vi "UPRcontroller_v00_basedonlsmv66.vi"() -> ()   [LabVIEW 2015] (continued)
                            n907 = call "eraseCI_img.vi"() -> ()  [unwired: 12 in]
                            n908 = call "eraseAI_img.vi"() -> ()  [unwired: 12 in]
                          }
                          frame "Lifetime (scan)" {
                            n909 = disable-structure shown="Disabled" {
                              disable-tunnel: w3434 -> [w3435 _]
                              frame Disabled {
                                n910 = stacked-sequence {
                                tunnel: w3435 -> [_ _ w3449 _ _]
                                frame #0 {
                                n911 = disable-structure shown="Disabled" {
                                frame Disabled {
                                n912 = call "stoperaseCI.vi"() -> ()  [unwired: 12 in]
                                n913 = call "stoperaseDO_img.vi"() -> ()  [unwired: 12 in]
                                n914 = call "stoperaseAO_img.vi"() -> ()  [unwired: 12 in]
                                n915 = call "stoperaseAI_img.vi"() -> ()  [unwired: 12 in]
                                }
                                frame Enabled {
                                }
                                }
                                }
                                frame #1 {
                                n916 = disable-structure shown="Disabled" {
                                frame Disabled {
                                n917 = local read "Acquisition time"() -> (w3439:i32)
                                n918 = call "collect_allLT_img.vi"() -> ("counts"=w3441:i32)  [unwired: 1 out]
                                n919 = local read "counts"() -> (w3442:i32)
                                n920 = Add(x=w3442, y=w3441) -> (x+y=w3440:i32)
                                "counts" <- w3440
                                n921 = Divide(x=w3440, y=w3439) -> (x/y=w3438:dbl)
                                n922 = Multiply(x=1000.0, y=w3438) -> (x*y=w3437:dbl)
                                n923 = local write "Avg Counts/s"(w3437) -> ()
                                }
                                frame Enabled {
                                }
                                }
                                }
                                frame #2 {
                                w3445 = u16 0 items=["Stream to disk", "Post process", "real time process"] ("Ring")
                                n924 = local read "T3R Data processing"() -> (w3444:u16)
                                n925 = local read "save\ndata"() -> (w3447:bool)
                                n926 = Equal?(x=w3444, y=w3445) -> (x = y?=w3443:bool)
                                n927 = Not(x=w3443) -> (.not. x?=w3448:bool)
                                n928 = And(x=w3447, y=w3448) -> (x .and. y?=w3446:bool)
                                n929 = case shown="True" w3446 {
                                tunnel: w3449 -> [_ w3451]
                                frame False {
                                }
                                frame True {
                                n930 = local read "filename prefix"() -> (w3452:string)
                                n931 = local read "data dir"() -> (w3457:path)
                                n932 = call "2pparameters.vi"("command"="get") -> ("params out"=w3472:T12)  [unwired: 1 in]
                                n933 = call "generatedatafilename.vi"("timestamp"=w3451, "filename prefix in"=w3452) -> ("full-filename"=w3450:string)
                                n934 = Unbundle By Name(w3472) -> ("srate"=w3470:sgl, "sAOxy"=w3469:i32, "Xpixels Img"=w3467:i32, "Ypixels Img"=w3465:i32)
                                n935 = Concatenate Strings(w3450, ".lvpt3img" ("string")) -> (w3455:string)
                                n936 = Build Path(base path=w3457, name or relative path=w3455) -> (appended path=w3454:path)
                                n937 = To Unsigned Long Integer(number=w3470) -> (unsigned 32bit integer=w3471:u32)
                                n938 = To Unsigned Long Integer(number=w3469) -> (unsigned 32bit integer=w3468:u32)
                                n939 = To Unsigned Long Integer(number=w3467) -> (unsigned 32bit integer=w3466:u32)
                                n940 = To Unsigned Long Integer(number=w3465) -> (unsigned 32bit integer=w3464:u32)
                                n941 = call "PH-temp-raw.vi"("command"="get") -> ("array out"=w3463:u32[])  [unwired: 1 in]
                                n942 = Build Array (concatenate)(w3471, w3468, w3466, w3464, w3463) -> (w3462:u32[])
                                n943 = Open/Create/Replace File(file path (use dialog)=w3454, operation (0:open)=T9."replace or create") -> (refnum out=w3461:refnum<file>, error out=w3460:errorcluster)  [unwired: 4 in, 1 out]
                                n944 = Write to Binary File(file (use dialog)=w3461, data=w3462, error in=w3460, 5:FALSE ("prepend array or string size? (T)")) -> (refnum out=w3458:refnum<file>, error out=w3459:errorcluster)  [unwired: 2 in, 1 out]
                                n945 = Close File(refnum=w3458, error in=w3459) -> ()  [unwired: 2 out]
                                }
                                }
                                n946 = call "stoperaseLT_img.vi"() -> ()  [unwired: 1 in]
                                }
                                frame #3 {
                                w3478 = u16 1 items=["Stream to disk", "Post process", "real time process"] ("Ring")
                                n947 = local read "T3R Data processing"() -> (w3477:u16)
                                n948 = Equal?(x=w3477, y=w3478) -> (x = y?=w3476:bool)
                                n949 = case shown="True" w3476 {
                                frame False {
                                }
                                frame True {
                                # "intensity"
                                # "lifetime"
                                # "intensity"
                                n950 = property on="img_CH1" class="IntGraph (strict)"() -> ("Value"=w3491:sgl[][])  [unwired: 2 in, 2 out]
                                n951 = Array Max & Min(array=w3491) -> (max value=w3492:sgl)  [unwired: 3 out]
                                n952 = local read "lineshift"() -> (w3479:i32)
                                n953 = local read "min phot"() -> (w3493:u32)
                                n954 = To Unsigned Long Integer(number=w3492) -> (unsigned 32bit integer=w3495:u32)
                                n955 = local read "counts"() -> (w3481:i32)
                                n956 = call "wrapcutlifetime.vi"("lineshift"=w3479) -> ("pt3img"=w3490:u16[][], "lifetimes"=w3488:sgl[][], "okay"=w3483:bool, "# of frames"=w3480:i32)
                                "frames recorded" <- w3480
                                n957 = Greater?(x=w3493, y=w3495) -> (0:w3494:bool)
                                n958 = Quotient & Remainder(x=w3481, y=w3480) -> (floor(x/y)=w3482:i32)  [unwired: 1 out]
                                n959 = Transpose 2D Array(2D array=w3490) -> (transposed array=w3484:u16[][])
                                n960 = Transpose 2D Array(2D array=w3488) -> (transposed array=w3489:sgl[][])
                                n961 = And(x=w3494, y=w3483) -> (x .and. y?=w3496:bool)
                                n962 = local write "img_CH2"(w3489) -> ()
                                n963 = local write "photons/frame"(w3482) -> ()
                                n964 = Array Max & Min(array=w3484) -> (max value=w3485:u16)  [unwired: 3 out]
                                n965 = To Single Precision Float(number=w3484) -> (single precision float=w3487:sgl[][])
                                n966 = case shown="True" w3496 {
                                tunnel: w3495 -> [_ w3500]
                                frame False {
                                }
                                frame True {
                                n967 = Quotient & Remainder(x=w3500, y=u32 2 ("min phot")) -> (floor(x/y)=w3499:u32)  [unwired: 1 out]
                                n968 = Max & Min(x=w3499, y=u32 5) -> (max(x,y)=w3498:u32)  [unwired: 1 out]
                                n969 = local write "min phot"(w3498) -> ()
                                }
                                }
                                n970 = To Double Precision Float(number=w3485) -> (double precision float=w3486:dbl)
                                n971 = local write "img_CH1"(w3487) -> ()
                                n972 = property on="img_CH1" class="IntGraph (strict)"("ZScale.Maximum"=w3486) -> ()  [unwired: 2 in, 2 out]
                                }
                                }
                                }
                                frame #4 {
                                w3504 = u16 1 items=["Stream to disk", "Post process", "real time process"] ("Ring")
                                n973 = local read "T3R Data processing"() -> (w3503:u16)
                                n974 = Equal?(x=w3503, y=w3504) -> (x = y?=w3502:bool)
                                n975 = case shown="False" w3502 {
                                frame False {
                                # "intensity"
                                n976 = local read "Current Average"() -> (w3509:sgl)
                                n977 = local read "image2list"() -> (w3505:u16)
                                n978 = local read "image1list"() -> (w3506:u16)
                                n979 = call "dattoimage.vi"("image2list"=w3505, "Current Average"=w3509, "image1list"=w3506) -> ("image 1 array out"=w3508:sgl[][])  [unwired: 1 out]
                                n980 = Transpose 2D Array(2D array=w3508) -> (transposed array=w3507:sgl[][])
                                n981 = local write "img_CH2"(w3507) -> ()
                                }
                                frame True {
                                }
                                }
                                }
                                }
                              }
                              frame Enabled {
                              }
                            }
                          }
                        }
                        n982 = local write "64bit disabled"(TRUE ("64bit disabled")) -> ()
                      }
                      frame #9 {
                        # "Reset the AO values after scanning to a known state (possibly source of delay after pressing stop)"
                        n983 = call "2pparameters.vi"("command"="get") -> ("params out"=w3514:T12)  [unwired: 1 in]
                        n984 = Unbundle By Name(w3514) -> ("auto OD"=w3513:bool, "autoshutter"=w3511:bool, "aAS"=w3510:u32[])
                        n985 = case shown="True" w3513 {
                          frame False {
                          }
                          frame True {
                            n986 = call "configuration.vi"("command"="get") -> ("config out"=w3519:T14)  [unwired: 2 in, 1 out]
                            n987 = call "2pparameters.vi"("command"="get") -> ("params out"=w3522:T12)  [unwired: 1 in]
                            n988 = Unbundle By Name(w3519) -> ("image OD"=w3517:u16)
                            n989 = Unbundle By Name(w3522) -> ("ODfilt"=w3518:u16)
                            n990 = call "filterwheelcontrol_nothorlabslib.vi"("Current OD filt"=w3517, "New ODfilt"=w3518) -> ()  [unwired: 1 in]
                          }
                        }
                        n991 = case shown="True" w3511 {
                          tunnel: w3510 -> [_ w3515]
                          frame False {
                          }
                          frame True {
                            n992 = call "shuttercontrol_multi.vi"("Autoshutter Chans"=w3515, "command"="close") -> ()  [unwired: 1 in, 1 out]
                          }
                        }
                        n993 = disable-structure shown="Disabled" {
                          frame Disabled {
                            # "<- possible source of delay"
                            n994 = call "reset AO_DO_v3.vi"() -> ()  [unwired: 12 in]
                          }
                          frame Disabled {
                            # "<- possible source of delay"
                            n995 = call "reset AO_DO_v3.vi"() -> ()  [unwired: 12 in]
                          }
                          frame Enabled {
                          }
                        }
                        n996 = flat-sequence {
                          frame #0 {
                            n997 = call "reset AO_DO_v3.vi"() -> ()  [unwired: 12 in]
                          }
                          frame #1 {
                            n998 = call "stoperaseCI.vi"() -> ()  [unwired: 12 in]
                            n999 = call "stoperaseDO_img.vi"() -> ()  [unwired: 12 in]
                            n1000 = call "stoperaseAO_img.vi"() -> ()  [unwired: 12 in]
                            n1001 = call "stoperaseAI_img.vi"() -> ()  [unwired: 12 in]
                          }
                        }
                      }
                      frame #10 {
                        # "CI: counter input (for photon counting)"
                        # "If waveform determined scan... separates out scanning waveforms from 'waveform generation' waveforms"
                        n1002 = stacked-sequence {
                          tunnel: w3536 -> [w3539 _ _ _ _ _]
                          tunnel: w3535 -> [w3538 _ _ _ _ _]
                          tunnel: w3534 -> [w3537 _ _ _ _ _]
                          tunnel: w3533 -> [_ w3588 _ _ _ _]
                          tunnel: w3532 -> [_ w3587 w3642 w3761 _ _]
                          tunnel: w3531 -> [_ w3586 w3641 w3760 _ _]
                          tunnel: w3530 -> [_ _ w3640 _ _ _]
                          tunnel: w3529 -> [_ _ w3639 _ _ _]
                          tunnel: w3528 -> [_ _ _ w3759 _ _]
                          tunnel: w3527 -> [_ _ _ w3758 _ _]
                          tunnel: w3526 -> [_ _ w3637 _ _ _]
                          tunnel: w3525 -> [_ _ w3636 _ _ _]
                          tunnel: w3524 -> [_ _ _ w3756 _ _]
                          tunnel: w3523 -> [_ _ _ w3755 _ _]
                          frame #0 {
                            # "Whether X galvo was added"
                            n1003 = case shown="True" w3539 {
                              tunnel: w3538 -> [_ w3561]
                              tunnel: w3537 -> [_ w3560]
                              frame True {
                                # "If added, remove it from wf parameters and add it to wave forms AO"
                                n1004 = stacked-sequence {
                                seq-local: [w3540 _ _] -> [_ w3552 w3557]
                                frame #0 {
                                n1005 = call "configuration.vi"("command"="get") -> ("config out"=w3546:T14)  [unwired: 2 in, 1 out]
                                n1006 = Unbundle By Name(w3546) -> ("Voltage to Xgalvo"=w3543:i32)
                                n1007 = call "2pparameters.vi"("command"="get") -> ("params out"=w3544:T12)  [unwired: 1 in]
                                n1008 = in-place {
                                in-place-border: w3543 -> [w3551]
                                in-place-border: [w3548] -> w3540
                                n1009 = in-place-cluster #9(w3544) -> ("aAO"=w3550:u32[])
                                n1010 = call "remove channel from active arrayv2.vi"("line array in"=w3550, "line to remove"=w3551) -> ("line array out"=w3549:u32[], "index"=w3548:i32)  [unwired: 1 out]
                                n1011 = in-place-cluster #9("aAO"=w3549) -> (w3541:T12)
                                }
                                n1012 = call "2pparameters.vi"("Params in"=w3541, "command"="set") -> ()  [unwired: 1 out]
                                }
                                frame #1 {
                                n1013 = call "waveformparamsv2.vi"("command"="rem AO", "index"=w3552) -> ()  [unwired: 3 in, 3 out]
                                }
                                frame #2 {
                                n1014 = call "waveformsAObuffer.vi"("command"="get") -> ("AO wf out"=w3558:waveform(dbl)[])  [unwired: 1 in]
                                n1015 = Delete From Array(array=w3558, length=1, index=w3557) -> (array with subset deleted=w3554:waveform(dbl)[])  [unwired: 1 out]
                                n1016 = call "waveformsAObuffer.vi"("AO wf in"=w3554, "command"="set") -> ()  [unwired: 1 out]
                                }
                                }
                              }
                              frame False {
                                # "If false, get it from AO parameters"
                                n1017 = stacked-sequence {
                                seq-local: [w3562 _ _] -> [_ w3570 w3581]
                                tunnel: w3561 -> [_ w3569 _]
                                tunnel: w3560 -> [_ _ w3580]
                                frame #0 {
                                n1018 = call "configuration.vi"("command"="get") -> ("config out"=w3567:T14)  [unwired: 2 in, 1 out]
                                n1019 = Unbundle By Name(w3567) -> ("Voltage to Xgalvo"=w3563:i32)
                                n1020 = call "2pparameters.vi"("command"="get") -> ("params out"=w3566:T12)  [unwired: 1 in]
                                n1021 = Unbundle By Name(w3566) -> ("aAO"=w3564:u32[])
                                n1022 = Search 1D Array(1D array=w3564, element=w3563) -> (index of element=w3562:i32)  [unwired: 1 in]
                                }
                                frame #1 {
                                n1023 = call "waveformparamsv2.vi"("command"="get") -> ("Params out"=w3573:T17)  [unwired: 4 in, 2 out]
                                n1024 = in-place {
                                in-place-border: w3570 -> [w3577]
                                in-place-border: w3569 -> [w3576]
                                n1025 = in-place-cluster #10(w3573) -> ("AO parameters"=w3578:T18)
                                n1026 = in-place {
                                in-place-border: w3576 -> [w3579]
                                n1027 = in-place-array #11(w3578, w3577) -> ()  [unwired: 1 out]
                                n1028 = in-place-array #11(w3579) -> (w3575:T18)  [unwired: 1 out]
                                }
                                n1029 = in-place-cluster #10("AO parameters"=w3575) -> (w3571:T17)
                                }
                                n1030 = call "waveformparamsv2.vi"("command"="set", "Params in"=w3571) -> ()  [unwired: 3 in, 3 out]
                                }
                                frame #2 {
                                n1031 = call "waveformsAObuffer.vi"("command"="get") -> ("AO wf out"=w3584:waveform(dbl)[])  [unwired: 1 in]
                                n1032 = Replace Array Subset(array=w3584, new element=w3580, index=w3581) -> (w3582:waveform(dbl)[])
                                n1033 = call "waveformsAObuffer.vi"("AO wf in"=w3582, "command"="set") -> ()  [unwired: 1 out]
                                }
                                }
                              }
                            }
                          }
                          frame #1 {
                            # "same as last frame but for Y galvo waveform"
                            n1034 = case shown="True" w3588 {
                              tunnel: w3587 -> [_ w3610]
                              tunnel: w3586 -> [_ w3609]
                              frame True {
                                n1035 = stacked-sequence {
                                seq-local: [w3589 _ _] -> [_ w3601 w3606]
                                frame #0 {
                                n1036 = call "configuration.vi"("command"="get") -> ("config out"=w3595:T14)  [unwired: 2 in, 1 out]
                                n1037 = Unbundle By Name(w3595) -> ("Voltage to Ygalvo"=w3592:i32)
                                n1038 = call "2pparameters.vi"("command"="get") -> ("params out"=w3593:T12)  [unwired: 1 in]
                                n1039 = in-place {
                                in-place-border: w3592 -> [w3600]
                                in-place-border: [w3597] -> w3589
                                n1040 = in-place-cluster #12(w3593) -> ("aAO"=w3599:u32[])
                                n1041 = call "remove channel from active arrayv2.vi"("line array in"=w3599, "line to remove"=w3600) -> ("line array out"=w3598:u32[], "index"=w3597:i32)  [unwired: 1 out]
                                n1042 = in-place-cluster #12("aAO"=w3598) -> (w3590:T12)
                                }
                                n1043 = call "2pparameters.vi"("Params in"=w3590, "command"="set") -> ()  [unwired: 1 out]
                                }
                                frame #1 {
                                n1044 = call "waveformparamsv2.vi"("command"="rem AO", "index"=w3601) -> ()  [unwired: 3 in, 3 out]
                                }
                                frame #2 {
                                n1045 = call "waveformsAObuffer.vi"("command"="get") -> ("AO wf out"=w3607:waveform(dbl)[])  [unwired: 1 in]
                                n1046 = Delete From Array(array=w3607, length=1, index=w3606) -> (array with subset deleted=w3603:waveform(dbl)[])  [unwired: 1 out]
                                n1047 = call "waveformsAObuffer.vi"("AO wf in"=w3603, "command"="set") -> ()  [unwired: 1 out]
                                }
                                }
                              }
                              frame False {
                                n1048 = stacked-sequence {
                                seq-local: [w3611 _ _] -> [_ w3619 w3630]
                                tunnel: w3610 -> [_ w3618 _]
                                tunnel: w3609 -> [_ _ w3629]
                                frame #0 {
                                n1049 = call "configuration.vi"("command"="get") -> ("config out"=w3616:T14)  [unwired: 2 in, 1 out]
                                n1050 = Unbundle By Name(w3616) -> ("Voltage to Ygalvo"=w3612:i32)
                                n1051 = call "2pparameters.vi"("command"="get") -> ("params out"=w3615:T12)  [unwired: 1 in]
                                n1052 = Unbundle By Name(w3615) -> ("aAO"=w3613:u32[])
                                n1053 = Search 1D Array(1D array=w3613, element=w3612) -> (index of element=w3611:i32)  [unwired: 1 in]
                                }
                                frame #1 {
                                n1054 = call "waveformparamsv2.vi"("command"="get") -> ("Params out"=w3622:T17)  [unwired: 4 in, 2 out]
                                n1055 = in-place {
                                in-place-border: w3619 -> [w3626]
                                in-place-border: w3618 -> [w3625]
                                n1056 = in-place-cluster #13(w3622) -> ("AO parameters"=w3627:T18)
                                n1057 = in-place {
                                in-place-border: w3625 -> [w3628]
                                n1058 = in-place-array #14(w3627, w3626) -> ()  [unwired: 1 out]
                                n1059 = in-place-array #14(w3628) -> (w3624:T18)  [unwired: 1 out]
                                }
                                n1060 = in-place-cluster #13("AO parameters"=w3624) -> (w3620:T17)
                                }
                                n1061 = call "waveformparamsv2.vi"("command"="set", "Params in"=w3620) -> ()  [unwired: 3 in, 3 out]
                                }
                                frame #2 {
                                n1062 = call "waveformsAObuffer.vi"("command"="get") -> ("AO wf out"=w3633:waveform(dbl)[])  [unwired: 1 in]
                                n1063 = Replace Array Subset(array=w3633, new element=w3629, index=w3630) -> (w3631:waveform(dbl)[])
                                n1064 = call "waveformsAObuffer.vi"("AO wf in"=w3631, "command"="set") -> ()  [unwired: 1 out]
                                }
                                }
                              }
                            }
                          }
                          frame #2 {
                            # "correctly output the  waveforms affected by both (autoshutter) and (waveform determined)"
                            n1065 = Build Array(w3637, w3636) -> (w3635:bool[])
                            n1066 = Boolean Array To Number(Boolean array=w3635) -> (number=w3638:u32)
                            n1067 = case shown="0" w3638 {
                              tunnel: w3642 -> [_ _ w3702]
                              tunnel: w3641 -> [_ _ w3701]
                              tunnel: w3640 -> [_ w3672 w3699]
                              tunnel: w3639 -> [_ w3671 w3700]
                              frame 1, Default {
                                n1068 = stacked-sequence {
                                seq-local: [w3645 _ _] -> [_ w3657 w3662]
                                frame #0 {
                                # "Remove autoshutter channel from DO list in 2p parameters"
                                n1069 = call "2pparameters.vi"("command"="get") -> ("params out"=w3644:T12)  [unwired: 1 in]
                                n1070 = Unbundle By Name(w3644) -> ("aAS"=w3643:u32[])
                                n1071 = for {
                                tunnel: [w3651] -> w3645 mode=indexing
                                tunnel: w3643 -> [w3649] mode=indexing
                                shift-right: [w3652] -> w3646
                                shift-left: w3644 -> [w3650]
                                n1072 = in-place {
                                in-place-border: w3649 -> [w3656]
                                in-place-border: [w3653] -> w3651
                                n1073 = in-place-cluster #15(w3650) -> ("aDO"=w3655:u32[])
                                n1074 = call "remove channel from active arrayv2.vi"("line array in"=w3655, "line to remove"=w3656) -> ("line array out"=w3654:u32[], "index"=w3653:i32)  [unwired: 1 out]
                                n1075 = in-place-cluster #15("aDO"=w3654) -> (w3652:T12)
                                }
                                }
                                n1076 = call "2pparameters.vi"("Params in"=w3646, "command"="set") -> ()  [unwired: 1 out]
                                }
                                frame #1 {
                                n1077 = for {
                                tunnel: w3657 -> [w3658] mode=indexing
                                n1078 = call "waveformparamsv2.vi"("command"="rem DO", "index"=w3658) -> ()  [unwired: 3 in, 3 out]
                                }
                                }
                                frame #2 {
                                # "sort so it removes the last elements first\nand does not mess up the order"
                                # "Remove waveforms of autoshutter channels from wave forms DO"
                                n1079 = call "waveformsDObuffer.vi"("command"="get") -> ("DO wf out"=w3665:digitalwaveform[])  [unwired: 1 in]
                                n1080 = Sort 1D Array(array=w3662) -> (sorted array=w3661:i32[])
                                n1081 = Reverse 1D Array(array=w3661) -> (reversed array=w3660:i32[])
                                n1082 = for {
                                tunnel: w3660 -> [w3667] mode=indexing
                                shift-right: [w3668] -> w3663
                                shift-left: w3665 -> [w3670]
                                n1083 = Delete From Array(array=w3670, length=1, index=w3667) -> (array with subset deleted=w3668:digitalwaveform[])  [unwired: 1 out]
                                }
                                n1084 = call "waveformsDObuffer.vi"("DO wf in"=w3663, "command"="set") -> ()  [unwired: 1 out]
                                }
                                }
                              }
                              frame 2 {
                                n1085 = stacked-sequence {
                                tunnel: w3672 -> [_ w3686 _]
                                tunnel: w3671 -> [_ _ w3693]
                                frame #0 {
                                # "add autoshutter channels to digital out"
                                n1086 = disable-structure shown="Disabled" {
                                frame Disabled {
                                n1087 = call "configuration.vi"("command"="get") -> ("config out"=w3678:T14)  [unwired: 2 in, 1 out]
                                n1088 = Unbundle By Name(w3678) -> ()  [unwired: 1 out]
                                }
                                frame Enabled {
                                }
                                }
                                n1089 = call "2pparameters.vi"("command"="get") -> ("params out"=w3674:T12)  [unwired: 1 in]
                                n1090 = Unbundle By Name(w3674) -> ("aAS"=w3673:u32[])
                                n1091 = in-place {
                                in-place-border: w3673 -> [w3680]
                                n1092 = in-place-cluster #16(w3674) -> ("aDO"=w3682:u32[])
                                n1093 = for {
                                shift-right: [w3684] -> w3681
                                shift-left: w3682 -> [w3685]
                                tunnel: w3680 -> [w3683] mode=indexing
                                n1094 = call "add channel to active arrayv2.vi"("line array in"=w3685, "line to add"=w3683) -> ("line array out"=w3684:u32[])  [unwired: 2 out]
                                }
                                n1095 = in-place-cluster #16("aDO"=w3681) -> (w3675:T12)
                                }
                                n1096 = call "2pparameters.vi"("Params in"=w3675, "command"="set") -> ()  [unwired: 1 out]
                                }
                                frame #1 {
                                # "Not sure the correct way to add multiple sets of parameters..."
                                # "add autoshutter waveforms to wf parameters v2"
                                n1097 = disable-structure shown="Disabled" {
                                disable-tunnel: w3686 -> [w3688 _]
                                frame Disabled {
                                n1098 = for {
                                tunnel: w3688 -> [w3689] mode=indexing
                                n1099 = call "waveformparamsv2.vi"("command"="add DO", "add DO"=w3689) -> ()  [unwired: 3 in, 3 out]
                                }
                                }
                                frame Enabled {
                                }
                                }
                                n1100 = call "waveformparamsv2.vi"("command"="add DO", "add DO"=w3686) -> ()  [unwired: 3 in, 3 out]
                                }
                                frame #2 {
                                # "add autoshutter waveforms to wave forms DO"
                                n1101 = call "waveformsDObuffer.vi"("command"="get") -> ("DO wf out"=w3694:digitalwaveform[])  [unwired: 1 in]
                                n1102 = for {
                                tunnel: w3693 -> [w3697] mode=indexing
                                shift-right: [w3696] -> w3691
                                shift-left: w3694 -> [w3698]
                                n1103 = Build Array (concatenate)(w3698, w3697) -> (w3696:digitalwaveform[])
                                }
                                n1104 = call "waveformsDObuffer.vi"("DO wf in"=w3691, "command"="set") -> ()  [unwired: 1 out]
                                }
                                }
                              }
                              frame 0 {
                                n1105 = stacked-sequence {
                                seq-local: [w3704 _ _] -> [_ w3712 w3736]
                                tunnel: w3702 -> [_ _ _]
                                tunnel: w3701 -> [_ _ _]
                                tunnel: w3700 -> [_ _ w3735]
                                tunnel: w3699 -> [_ w3711 _]
                                frame #0 {
                                n1106 = call "2pparameters.vi"("command"="get") -> ("params out"=w3707:T12)  [unwired: 1 in]
                                n1107 = Unbundle By Name(w3707) -> ("aDO"=w3705:u32[], "aAS"=w3703:u32[])
                                n1108 = for {
                                tunnel: w3705 -> [w3710]
                                tunnel: [w3709] -> w3704 mode=indexing
                                tunnel: w3703 -> [w3708] mode=indexing
                                n1109 = Search 1D Array(1D array=w3710, element=w3708) -> (index of element=w3709:i32)  [unwired: 1 in]
                                }
                                }
                                frame #1 {
                                n1110 = call "2pparameters.vi"("command"="get") -> ("params out"=w3715:T12)  [unwired: 1 in]
                                n1111 = Unbundle By Name(w3715) -> ("wavdet"=w3713:bool, "autoshutter"=w3714:bool)
                                n1112 = case shown="True" w3714 {
                                tunnel: w3712 -> [_ w3719]
                                tunnel: w3713 -> [_ w3718]
                                tunnel: w3711 -> [_ w3717]
                                frame False {
                                }
                                frame True {
                                n1113 = case shown="False" w3718 {
                                tunnel: w3719 -> [w3721 _]
                                tunnel: w3717 -> [w3720 _]
                                frame False {
                                # "Replace autoshutter channel DO waveforms with those that were generated from autoshutter."
                                n1114 = call "waveformparamsv2.vi"("command"="get") -> ("Params out"=w3724:T17)  [unwired: 4 in, 2 out]
                                n1115 = in-place {
                                in-place-border: w3721 -> [w3728]
                                in-place-border: w3720 -> [w3726]
                                n1116 = in-place-cluster #17(w3724) -> ("DO parameters"=w3729:T20)
                                n1117 = for {
                                tunnel: w3728 -> [w3732] mode=indexing
                                tunnel: w3726 -> [w3730] mode=indexing
                                shift-right: [w3731] -> w3727
                                shift-left: w3729 -> [w3733]
                                n1118 = in-place {
                                in-place-border: w3730 -> [w3734]
                                n1119 = in-place-array #18(w3733, w3732) -> ()  [unwired: 1 out]
                                n1120 = in-place-array #18(w3734) -> (w3731:T20)  [unwired: 1 out]
                                }
                                }
                                n1121 = in-place-cluster #17("DO parameters"=w3727) -> (w3722:T17)
                                }
                                n1122 = call "waveformparamsv2.vi"("command"="set", "Params in"=w3722) -> ()  [unwired: 3 in, 3 out]
                                }
                                frame True {
                                }
                                }
                                }
                                }
                                }
                                frame #2 {
                                n1123 = call "2pparameters.vi"("command"="get") -> ("params out"=w3739:T12)  [unwired: 1 in]
                                n1124 = Unbundle By Name(w3739) -> ("wavdet"=w3737:bool, "autoshutter"=w3738:bool)
                                n1125 = case shown="True" w3738 {
                                tunnel: w3736 -> [_ w3743]
                                tunnel: w3737 -> [_ w3742]
                                tunnel: w3735 -> [_ w3741]
                                frame False {
                                }
                                frame True {
                                n1126 = case shown="False" w3742 {
                                tunnel: w3743 -> [w3745 _]
                                tunnel: w3741 -> [w3744 _]
                                frame False {
                                # "replace autoshutter channels of waveforms DO with autoshutter waveforms"
                                n1127 = call "waveformsDObuffer.vi"("command"="get") -> ("DO wf out"=w3747:digitalwaveform[])  [unwired: 1 in]
                                n1128 = for {
                                tunnel: w3745 -> [w3751] mode=indexing
                                tunnel: w3744 -> [w3750] mode=indexing
                                shift-right: [w3753] -> w3749
                                shift-left: w3747 -> [w3752]
                                n1129 = Replace Array Subset(array=w3752, new element=w3750, index=w3751) -> (w3753:digitalwaveform[])
                                }
                                n1130 = call "waveformsDObuffer.vi"("DO wf in"=w3749, "command"="set") -> ()  [unwired: 1 out]
                                }
                                frame True {
                                }
                                }
                                }
                                }
                                }
                                }
                              }
                            }
                          }
                          frame #3 {
                            # "Same thing for LT timestamp (?what is that?)"
                            n1131 = Build Array(w3756, w3755) -> (w3757:bool[])
                            n1132 = Boolean Array To Number(Boolean array=w3757) -> (number=w3754:u32)
                            n1133 = case shown="0" w3754 {
                              tunnel: w3761 -> [_ _ w3804]
                              tunnel: w3760 -> [_ _ w3803]
                              tunnel: w3759 -> [_ w3783 w3801]
                              tunnel: w3758 -> [_ w3782 w3802]
                              frame 1, Default {
                                n1134 = stacked-sequence {
                                seq-local: [w3762 _ _] -> [_ w3774 w3779]
                                frame #0 {
                                n1135 = call "configuration.vi"("command"="get") -> ("config out"=w3768:T14)  [unwired: 2 in, 1 out]
                                n1136 = Unbundle By Name(w3768) -> ("LT timestamp"=w3765:u32)
                                n1137 = call "2pparameters.vi"("command"="get") -> ("params out"=w3766:T12)  [unwired: 1 in]
                                n1138 = in-place {
                                in-place-border: w3765 -> [w3773]
                                in-place-border: [w3770] -> w3762
                                n1139 = in-place-cluster #19(w3766) -> ("aDO"=w3772:u32[])
                                n1140 = call "remove channel from active arrayv2.vi"("line array in"=w3772, "line to remove"=w3773) -> ("line array out"=w3771:u32[], "index"=w3770:i32)  [unwired: 1 out]
                                n1141 = in-place-cluster #19("aDO"=w3771) -> (w3763:T12)
                                }
                                n1142 = call "2pparameters.vi"("Params in"=w3763, "command"="set") -> ()  [unwired: 1 out]
                                }
                                frame #1 {
                                n1143 = call "waveformparamsv2.vi"("command"="rem DO", "index"=w3774) -> ()  [unwired: 3 in, 3 out]
                                }
                                frame #2 {
                                n1144 = call "waveformsDObuffer.vi"("command"="get") -> ("DO wf out"=w3780:digitalwaveform[])  [unwired: 1 in]
                                n1145 = Delete From Array(array=w3780, length=1, index=w3779) -> (array with subset deleted=w3776:digitalwaveform[])  [unwired: 1 out]
                                n1146 = call "waveformsDObuffer.vi"("DO wf in"=w3776, "command"="set") -> ()  [unwired: 1 out]
                                }
                                }
                              }
                              frame 2 {
                                n1147 = stacked-sequence {
                                tunnel: w3783 -> [_ _ w3796]
                                tunnel: w3782 -> [_ w3794 _]
                                frame #0 {
                                n1148 = call "configuration.vi"("command"="get") -> ("config out"=w3785:T14)  [unwired: 2 in, 1 out]
                                n1149 = Unbundle By Name(w3785) -> ("LT timestamp"=w3784:u32)
                                n1150 = call "2pparameters.vi"("command"="get") -> ("params out"=w3789:T12)  [unwired: 1 in]
                                n1151 = in-place {
                                in-place-border: w3784 -> [w3793]
                                n1152 = in-place-cluster #20(w3789) -> ("aDO"=w3792:u32[])
                                n1153 = call "add channel to active arrayv2.vi"("line array in"=w3792, "line to add"=w3793) -> ("line array out"=w3791:u32[])  [unwired: 2 out]
                                n1154 = in-place-cluster #20("aDO"=w3791) -> (w3787:T12)
                                }
                                n1155 = call "2pparameters.vi"("Params in"=w3787, "command"="set") -> ()  [unwired: 1 out]
                                }
                                frame #1 {
                                n1156 = call "waveformparamsv2.vi"("command"="add DO", "add DO"=w3794) -> ()  [unwired: 3 in, 3 out]
                                }
                                frame #2 {
                                n1157 = call "waveformsDObuffer.vi"("command"="get") -> ("DO wf out"=w3799:digitalwaveform[])  [unwired: 1 in]
                                n1158 = Build Array (concatenate)(w3799, w3796) -> (w3798:digitalwaveform[])
                                n1159 = call "waveformsDObuffer.vi"("DO wf in"=w3798, "command"="set") -> ()  [unwired: 1 out]
                                }
                                }
                              }
                              frame 0 {
                                n1160 = stacked-sequence {
                                seq-local: [w3805 _ _] -> [_ w3815 w3832]
                                tunnel: w3804 -> [_ _ _]
                                tunnel: w3803 -> [_ _ _]
                                tunnel: w3802 -> [_ w3812 _]
                                tunnel: w3801 -> [_ _ w3831]
                                frame #0 {
                                n1161 = call "configuration.vi"("command"="get") -> ("config out"=w3810:T14)  [unwired: 2 in, 1 out]
                                n1162 = Unbundle By Name(w3810) -> ("LT timestamp"=w3806:u32)
                                n1163 = call "2pparameters.vi"("command"="get") -> ("params out"=w3809:T12)  [unwired: 1 in]
                                n1164 = Unbundle By Name(w3809) -> ("aDO"=w3807:u32[])
                                n1165 = Search 1D Array(1D array=w3807, element=w3806) -> (index of element=w3805:i32)  [unwired: 1 in]
                                }
                                frame #1 {
                                n1166 = local read "Measurement"() -> (w3814:T4)
                                n1167 = To Unsigned Long Integer(number=w3814) -> (unsigned 32bit integer=w3813:u32)
                                n1168 = case shown="5..7" w3813 {
                                tunnel: w3815 -> [_ w3819]
                                tunnel: w3812 -> [_ w3816]
                                frame 0..4, Default {
                                }
                                frame 5..7 {
                                n1169 = Index Array(array=w3816, index=0) -> (element=w3817:T21)
                                n1170 = call "waveformparamsv2.vi"("command"="get") -> ("Params out"=w3822:T17)  [unwired: 4 in, 2 out]
                                n1171 = in-place {
                                in-place-border: w3819 -> [w3826]
                                in-place-border: w3817 -> [w3824]
                                n1172 = in-place-cluster #21(w3822) -> ("DO parameters"=w3827:T20)
                                n1173 = in-place {
                                in-place-border: w3824 -> [w3828]
                                n1174 = in-place-array #22(w3827, w3826) -> ()  [unwired: 1 out]
                                n1175 = in-place-array #22(w3828) -> (w3825:T20)  [unwired: 1 out]
                                }
                                n1176 = in-place-cluster #21("DO parameters"=w3825) -> (w3820:T17)
                                }
                                n1177 = call "waveformparamsv2.vi"("command"="set", "Params in"=w3820) -> ()  [unwired: 3 in, 3 out]
                                }
                                }
                                }
                                frame #2 {
                                n1178 = local read "Measurement"() -> (w3830:T4)
                                n1179 = To Unsigned Long Integer(number=w3830) -> (unsigned 32bit integer=w3829:u32)
                                n1180 = case shown="5..7" w3829 {
                                tunnel: w3832 -> [_ w3836]
                                tunnel: w3831 -> [_ w3834]
                                frame 0..4, Default {
                                }
                                frame 5..7 {
                                n1181 = Index Array(array=w3834, index=0) -> (element=w3833:digitalwaveform)
                                n1182 = call "waveformsDObuffer.vi"("command"="get") -> ("DO wf out"=w3838:digitalwaveform[])  [unwired: 1 in]
                                n1183 = Replace Array Subset(array=w3838, new element=w3833, index=w3836) -> (w3840:digitalwaveform[])
                                n1184 = call "waveformsDObuffer.vi"("DO wf in"=w3840, "command"="set") -> ()  [unwired: 1 out]
                                }
                                }
                                }
                                }
                              }
                            }
                          }
                          frame #4 {
                            # "Looks like its updating the waveforms pallette with relevant info"
                            n1185 = call "Used AO lines.vi"() -> ("used AO names"=w3843:string[], "used AO lines"=w3841:tag[])  [unwired: 2 in]
                            n1186 = control-ref of="Analog Lines Plot"() -> (w3842:refnum<vi>)
                            n1187 = control-ref of="Digital Lines Plot"() -> (w3844:refnum<vi>)
                            n1188 = call "Used DO lines.vi"() -> ("used DO names"=w3845:string[], "used DO lines"=w3846:tag[])  [unwired: 2 in]
                            n1189 = local write "Analog Used Lines"(w3841) -> ()
                            n1190 = local write "Analog Used Names"(w3843) -> ()
                            n1191 = local write "Digital Used Lines"(w3846) -> ()
                            n1192 = local write "Digital Used Names"(w3845) -> ()
                            n1193 = call "prepDOWaveplot.vi"("DigitalGraph in"=w3844, "used DO names"=w3845) -> ()  [unwired: 1 in]
                            n1194 = call "prepAOWaveplot.vi"("WaveformGraph in"=w3842, "Analog Used Names"=w3843) -> ()  [unwired: 1 in]
                          }
                          frame #5 {
                            # "Could this be source of crashing?"
                            n1195 = local read "Meastab"() -> (w3861:enum32{"X-Y Image", "Linescan", "Timetrace"})
                            n1196 = property on="refwf" class="Ring (strict)"() -> ("RingText.Text"=w3858:string)  [unwired: 2 in, 2 out]
                            n1197 = case shown="\"Timetrace\"" w3861 {
                              tunnel: [w3863 w3864] -> w3862
                              frame "X-Y Image", Default {
                                n1198 = local read "Sampling rate"() -> (w3863:dbl)
                              }
                              frame "Timetrace" {
                                n1199 = local read "srateAODOtt"() -> (w3864:dbl)
                              }
                            }
                            n1200 = call "waveformsAObuffer.vi"("command"="get") -> ("AO wf out"=w3849:waveform(dbl)[])  [unwired: 1 in]
                            n1201 = local read "wavdet"() -> (w3859:bool)
                            n1202 = call "waveformsDObuffer.vi"("command"="get") -> ("DO wf out"=w3853:digitalwaveform[])  [unwired: 1 in]
                            n1203 = call "correctwaveformsizetemp.vi"("new sampling frequency (Hz)"=w3862, "start"=FALSE, "reference waveforms to"=w3858, "Analog waveforms in"=w3849, "stop"=TRUE, "Digital waveforms in"=w3853) -> ("analog wf out"=w3855:waveform(dbl)[], "Digital wf out"=w3857:digitalwaveform[], "measpoints"=w3860:i32)
                            n1204 = local write "Analog Lines Plot"(w3855) -> ()
                            n1205 = call "GetNumCamFramesv2.vi"("Digital Waveform Graph"=w3857) -> ("Numeric"=w3856:i32)  [unwired: 10 in]
                            n1206 = local write "Digital Lines Plot"(w3857) -> ()
                            n1207 = call "waveformsDObuffer.vi"("DO wf in"=w3857, "command"="set") -> ()  [unwired: 1 out]
                            n1208 = call "waveformsAObuffer.vi"("AO wf in"=w3855, "command"="set") -> ()  [unwired: 1 out]
                            n1209 = local write "Total Camera Frames"(w3856) -> ()
                            n1210 = case shown="True" w3859 {
                              tunnel: w3860 -> [_ w3865]
                              frame False {
                              }
                              frame True {
                                n1211 = local write "# of frames"(w3865) -> ()
                              }
                            }
                          }
                        }
                      }
                      frame #11 {
                        w3873 = FALSE ("Value (Signaling)")
                        # "Cleanup... saves parameters and timestamps to a file and closes the file to which TIFFs are saved"
                        n1212 = local read "save\ndata"() -> (w3866:bool)
                        n1213 = local read "save\ndata"() -> (w3867:bool)
                        n1214 = property on="Stop" class="Bool (strict)"("Visible"=FALSE, "DisabledEnum"=T8."Disabled" ("Disabled")) -> ()  [unwired: 2 in, 2 out]
                        n1215 = case shown="True" w3866 {
                          frame False {
                          }
                          frame True {
                            n1216 = call "closetiffs.vi"() -> ()  [unwired: 12 in]
                          }
                        }
                        n1217 = case shown="True" w3867 {
                          tunnel: w3868 -> [_ w3876]
                          frame False {
                          }
                          frame True {
                            n1218 = local read "filename prefix"() -> (w3874:string)
                            n1219 = local read "data dir"() -> (w3875:path)
                            n1220 = call "savetimestamps.vi"("timestamp"=w3876, "filename prefix in"=w3874, "data dir in"=w3875) -> ()  [unwired: 1 in]
                            n1221 = call "saveparams_andscanpattern.vi"("filename prefix in"=w3874, "data dir in"=w3875) -> ()  [unwired: 2 in]
                            n1222 = disable-structure shown="Disabled" {
                              disable-tunnel: w3875 -> [w3878 _]
                              disable-tunnel: w3874 -> [w3877 _]
                              frame Disabled {
                                n1223 = call "saveparams.vi"("filename prefix in"=w3877, "data dir in"=w3878) -> ()  [unwired: 2 in]
                              }
                              frame Enabled {
                              }
                            }
                          }
                        }
                        n1224 = property on="Start" class="Bool (strict)"("Visible"=TRUE, "DisabledEnum"=T8."Enabled" ("Disabled")) -> ()  [unwired: 2 in, 2 out]
                        n1225 = property on="Start" class="Bool (strict)"("Val(Sgnl)"=w3873) -> ()  [unwired: 2 in, 2 out]
                        n1226 = property on="Stop" class="Bool (strict)"("Val(Sgnl)"=w3873) -> ()  [unwired: 2 in, 2 out]
                      }
                      frame #12 {
                        w3882 = T24 2 items=["no dialog", "OK message", "continue or stop message", "OK message + warnings", "continue/stop + warnings"] ("type of dialog (OK msg:1)")
                        # "Error handling"
                        n1227 = call "displayerrors.vi"() -> ("error IO"=w3881:errorcluster)
                        n1228 = call <vilib>:"General Error Handler.vi"("type of dialog (OK msg:1)"=w3882, "error in (no error)"=w3881) -> ("error out"=w3880:errorcluster)  [unwired: 9 in, 4 out]
                        n1229 = call <vilib>:"Clear Errors.vi"("error in (no error)"=w3880) -> ("error out"=w3879:errorcluster)  [unwired: 5 in, 1 out]
                        n1230 = call "seterrors.vi"("error IO"=w3879) -> ()
                      }
                    }
                  }
                  frame "X-Y-Z-t movie" {
                    n1231 = call "2pparameters.vi"("command"="get") -> ("params out"=w3885:T12)  [unwired: 1 in]
                    n1232 = Bundle By Name(cluster=w3885, "type"="X-Y-Z-t movie") -> (w3883:T12)
                    n1233 = call "2pparameters.vi"("Params in"=w3883, "command"="set") -> ()  [unwired: 1 out]
                  }
                  frame "linescan" {
                    n1234 = call "2pparameters.vi"("command"="get") -> ("params out"=w3890:T12)  [unwired: 1 in]
                    n1235 = Bundle By Name(cluster=w3890, "type"="linescan") -> (w3892:T12)
                    n1236 = call "2pparameters.vi"("Params in"=w3892, "command"="set") -> ()  [unwired: 1 out]
                  }
                  frame "Timetrace", "Lifetime (contour)" {
                    n1237 = local read "ttt"() -> (w3893:T3)
                    n1238 = case shown="\"Point\", \"Resonant Ellipse\", \"freeform contour\", \"Fill Ellipse\", Default" w3893 {
                      selector: w3893 -> [_ w3894]
                      frame "Line" {
                      }
                      frame "Point", "Resonant Ellipse", "freeform contour", "Fill Ellipse", Default {
                        n1239 = stacked-sequence {
                          seq-local: [w3910 _ _ _ _ _ _ _ _ _ _] -> [_ _ w4858 _ _ w4873 w4940 _ _ w5322 _]
                          seq-local: [w3909 _ _ _ _ _ _ _ _ _ _] -> [_ _ _ _ _ _ _ _ w4987 _ _]
                          seq-local: [w3908 _ _ _ _ _ _ _ _ _ _] -> [_ _ _ _ _ _ _ _ w4986 _ _]
                          seq-local: [w3907 _ _ _ _ _ _ _ _ _ _] -> [_ _ _ _ _ _ _ _ w4989 _ _]
                          seq-local: [w3906 _ _ _ _ _ _ _ _ _ _] -> [_ _ _ _ _ _ _ _ w4985 _ _]
                          seq-local: [w3905 _ _ _ _ _ _ _ _ _ _] -> [_ _ _ _ _ _ _ _ w4984 _ _]
                          seq-local: [w3904 _ _ _ _ _ _ _ _ _ _] -> [_ _ _ _ _ _ _ _ w4988 _ _]
                          seq-local: [w3903 _ _ _ _ _ _ _ _ _ _] -> [_ _ _ _ _ _ _ _ w4983 _ _]
                          seq-local: [w3902 _ _ _ _ _ _ _ _ _ _] -> [_ _ _ _ _ _ _ _ w4982 _ _]
                          seq-local: [w3901 _ _ _ _ _ _ _ _ _ _] -> [_ _ _ _ _ _ _ _ w4977 _ _]
                          seq-local: [w3900 _ _ _ _ _ _ _ _ _ _] -> [_ _ _ _ _ _ _ _ w4976 _ _]
                          seq-local: [w3899 _ _ _ _ _ _ _ _ _ _] -> [_ _ _ _ _ _ _ _ w4981 _ _]
                          seq-local: [w3898 _ _ _ _ _ _ _ _ _ _] -> [_ _ _ _ _ _ _ _ w4980 _ _]
                          seq-local: [w3897 _ _ _ _ _ _ _ _ _ _] -> [_ _ _ _ _ _ _ _ w4979 _ _]
                          seq-local: [w3896 _ _ _ _ _ _ _ _ _ _] -> [_ _ _ _ _ _ _ _ w4978 _ _]
                          tunnel: w3894 -> [w3895 _ _ _ _ _ _ _ _ _ _]
                          frame #0 {
                            n1240 = Get Date/Time In Seconds() -> (seconds since 1Jan1904=w3912:timestamp)
                            n1241 = local read "save\ndata"() -> (w3911:bool)
                            n1242 = case shown="False" w3911 {
                              tunnel: w3912 -> [w3913 w3915]
                              tunnel: [w3913 w3914] -> w3910
                              frame False {
                              }
                              frame True {
                                n1243 = call "createdatafolder.vi"("timestamp in"=w3915) -> ("current data path"=w3916:path, "timestamp out"=w3914:timestamp)
                                n1244 = local write "data dir"(w3916) -> ()
                              }
                            }
                            n1245 = stacked-sequence {
                              tunnel: w3910 -> [w3923 _ _ _ _ _ _ _ _]
                              tunnel: [_ _ _ _ _ _ w4131 _ _] -> w3909
                              tunnel: [_ _ _ _ _ _ w4130 _ _] -> w3908
                              tunnel: [_ _ _ _ _ _ w4129 _ _] -> w3907
                              tunnel: [_ _ _ _ _ _ w4128 _ _] -> w3906
                              tunnel: [_ _ _ _ _ _ w4127 _ _] -> w3905
                              tunnel: [_ _ _ _ _ _ w4126 _ _] -> w3904
                              tunnel: [_ _ _ _ _ _ w4125 _ _] -> w3903
                              tunnel: [_ _ _ _ _ _ w4124 _ _] -> w3902
                              tunnel: [_ _ _ _ _ _ w4123 _ _] -> w3901
                              tunnel: [_ _ _ _ _ _ w4122 _ _] -> w3900
                              tunnel: [_ _ _ _ _ _ w4121 _ _] -> w3899
                              tunnel: [_ _ _ _ _ _ w4120 _ _] -> w3898
                              tunnel: [_ _ _ _ _ _ w4119 _ _] -> w3897
                              tunnel: [_ _ _ _ _ _ w4118 _ _] -> w3896
                              tunnel: w3895 -> [_ _ w3962 _ w4022 _ _ _ _]
                              frame #0 {
                                # "creates date and time string... housekeeping"
                                n1246 = local read "Auto Shutter Channels"() -> (w3917:i32[])
                                n1247 = Format Date/Time String(time format string (%c)="%Y%m%d", seconds (now)=w3923) -> (date/time string=w3922:string)  [unwired: 1 in]
                                n1248 = Format Date/Time String(time format string (%c)="%H%M%S", seconds (now)=w3923) -> (date/time string=w3921:string)  [unwired: 1 in]
                                n1249 = local write "graphtab"(T5."timetrace" ("graphtab")) -> ()
                                n1250 = local read "AI channels"() -> (w3927:i32[])
                                n1251 = local read "CI channels"() -> (w3928:i32[])
                                n1252 = property on="Stop" class="Bool (strict)"("Visible"=TRUE, "DisabledEnum"=T8."Enabled" ("Disabled")) -> ()  [unwired: 2 in, 2 out]
                                n1253 = property on="Start" class="Bool (strict)"("Visible"=FALSE, "DisabledEnum"=T8."Disabled and Grayed Out" ("Disabled")) -> ()  [unwired: 2 in, 2 out]
                                n1254 = call "2pparameters.vi"("command"="get") -> ("params out"=w3930:T12)  [unwired: 1 in]
                                n1255 = Bundle By Name(cluster=w3930, "aAI"=w3927, "aCI"=w3928, "type"="Timetrace", "date"=w3922, "time"=w3921, "aAS"=w3917) -> (w3929:T12)
                                n1256 = call "X-array-databuffer.vi"("command"=enum16{"get", "set", "clear", "append"}."clear") -> ()  [unwired: 3 in, 2 out]
                                n1257 = call "Y-array-databuffer.vi"("command"=enum16{"get", "set", "clear", "append"}."clear") -> ()  [unwired: 3 in, 2 out]
                                n1258 = call "2pparameters.vi"("Params in"=w3929, "command"="set") -> ()  [unwired: 1 out]
                                n1259 = call "CH1-1D-temp.vi"("command"=enum16{"get", "set", "clear", "append"}."clear") -> ()  [unwired: 3 in, 2 out]
                                n1260 = call "CH2-1D-temp.vi"("command"=enum16{"get", "set", "clear", "append"}."clear") -> ()  [unwired: 3 in, 2 out]
                                n1261 = call "allAI-temp.vi"("command"=enum16{"get", "set", "clear", "append"}."clear") -> ()  [unwired: 3 in, 2 out]
                              }
                              frame #1 {
                                # "graph list for type of data to aquire"
                                n1262 = call "configuration.vi"("command"="get") -> ("config out"=w3947:T14)  [unwired: 2 in, 1 out]
                                n1263 = Unbundle By Name(w3947) -> ("CI names"=w3948:string[], "AI names"=w3949:string[])
                                n1264 = call "2pparameters.vi"("command"="get") -> ("params out"=w3943:T12)  [unwired: 1 in]
                                n1265 = Unbundle By Name(w3943) -> ("aCI"=w3944:i32[], "aAI"=w3945:i32[])
                                n1266 = for {
                                tunnel: w3944 -> [w3959] mode=indexing
                                tunnel: w3948 -> [w3960]
                                tunnel: [w3958] -> w3950 mode=indexing
                                n1267 = Index Array(array=w3960, index=w3959) -> (element=w3958:string)
                                }
                                n1268 = for {
                                tunnel: w3945 -> [w3956] mode=indexing
                                tunnel: w3949 -> [w3957]
                                tunnel: [w3955] -> w3951 mode=indexing
                                n1269 = Index Array(array=w3957, index=w3956) -> (element=w3955:string)
                                }
                                n1270 = Build Array (concatenate)(w3950, w3951) -> (w3941:string[])
                                n1271 = for {
                                tunnel: w3941 -> [w3953] mode=indexing
                                tunnel: [w3952] -> w3940 mode=indexing
                                i -> [w3954]
                                n1272 = Bundle("String"=w3953, w3954) -> (w3952:cluster{"String":string, i32})  [unwired: 1 in]
                                }
                                n1273 = property on="graph1list" class="Ring (strict)"("StringsAndValues[]"=w3940) -> ()  [unwired: 2 in, 2 out]
                                n1274 = property on="graph2list" class="Ring (strict)"("StringsAndValues[]"=w3940) -> ()  [unwired: 2 in, 2 out]
                              }
                              frame #2 {
                                # "OD wheel... doesnt work in 64bit labview"
                                n1275 = call "2pparameters.vi"("command"="get") -> ("params out"=w3965:T12)  [unwired: 1 in]
                                n1276 = Unbundle By Name(w3965) -> ("auto OD"=w3963:bool, "autoshutter"=w3966:bool, "aAS"=w3961:u32[])
                                n1277 = case shown="True" w3963 {
                                tunnel: w3962 -> [_ w3967]
                                frame False {
                                }
                                frame True {
                                n1278 = case shown="\"Point\"" w3967 {
                                frame "Point" {
                                n1279 = call "configuration.vi"("command"="get") -> ("config out"=w3970:T14)  [unwired: 2 in, 1 out]
                                n1280 = Unbundle By Name(w3970) -> ("point OD"=w3971:u16)
                                n1281 = local read "ODfilt"() -> (w3968:u16)
                                n1282 = call "filterwheelcontrol_nothorlabslib.vi"("Current OD filt"=w3968, "New ODfilt"=w3971) -> ()  [unwired: 1 in]
                                }
                                frame "Resonant Ellipse", Default {
                                n1283 = call "configuration.vi"("command"="get") -> ("config out"=w3974:T14)  [unwired: 2 in, 1 out]
                                n1284 = Unbundle By Name(w3974) -> ("contour OD"=w3975:u16)
                                n1285 = local read "ODfilt"() -> (w3972:u16)
                                n1286 = call "filterwheelcontrol_nothorlabslib.vi"("Current OD filt"=w3972, "New ODfilt"=w3975) -> ()  [unwired: 1 in]
                                }
                                }
                                }
                                }
                                n1287 = case shown="True" w3966 {
                                tunnel: w3961 -> [_ w3976]
                                frame False {
                                }
                                frame True {
                                n1288 = call "shuttercontrol_multi.vi"("Autoshutter Chans"=w3976, "command"="close") -> ()  [unwired: 1 in, 1 out]
                                }
                                }
